vi "SeqMgr.Sequence Load, Check Lines for Sourcing Other Files.vi"(7 "Search Folders":path[](array[path]), 8 "error in (no error)":errorcluster, 10 "Parent Scripts":path[](array[path]), 11 "Lines In":string[](array[string])) -> (0 "error out":errorcluster, 3 "Lines Out":string[](array[string]))   [LabVIEW 2024, in "EQMF.lvlib" / "SeqMgr.lvlib"]
uses:
  SeqMgr.lvlib
  <vilib>/Utility/error.llb/Trim Whitespace One-Sided.vi
  Files/File Utils.lvlib
  Strings/String Utils.lvlib
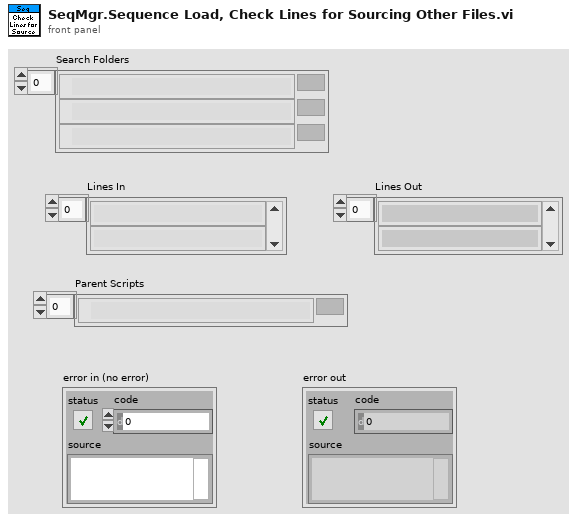
[diagram p1: front panel]
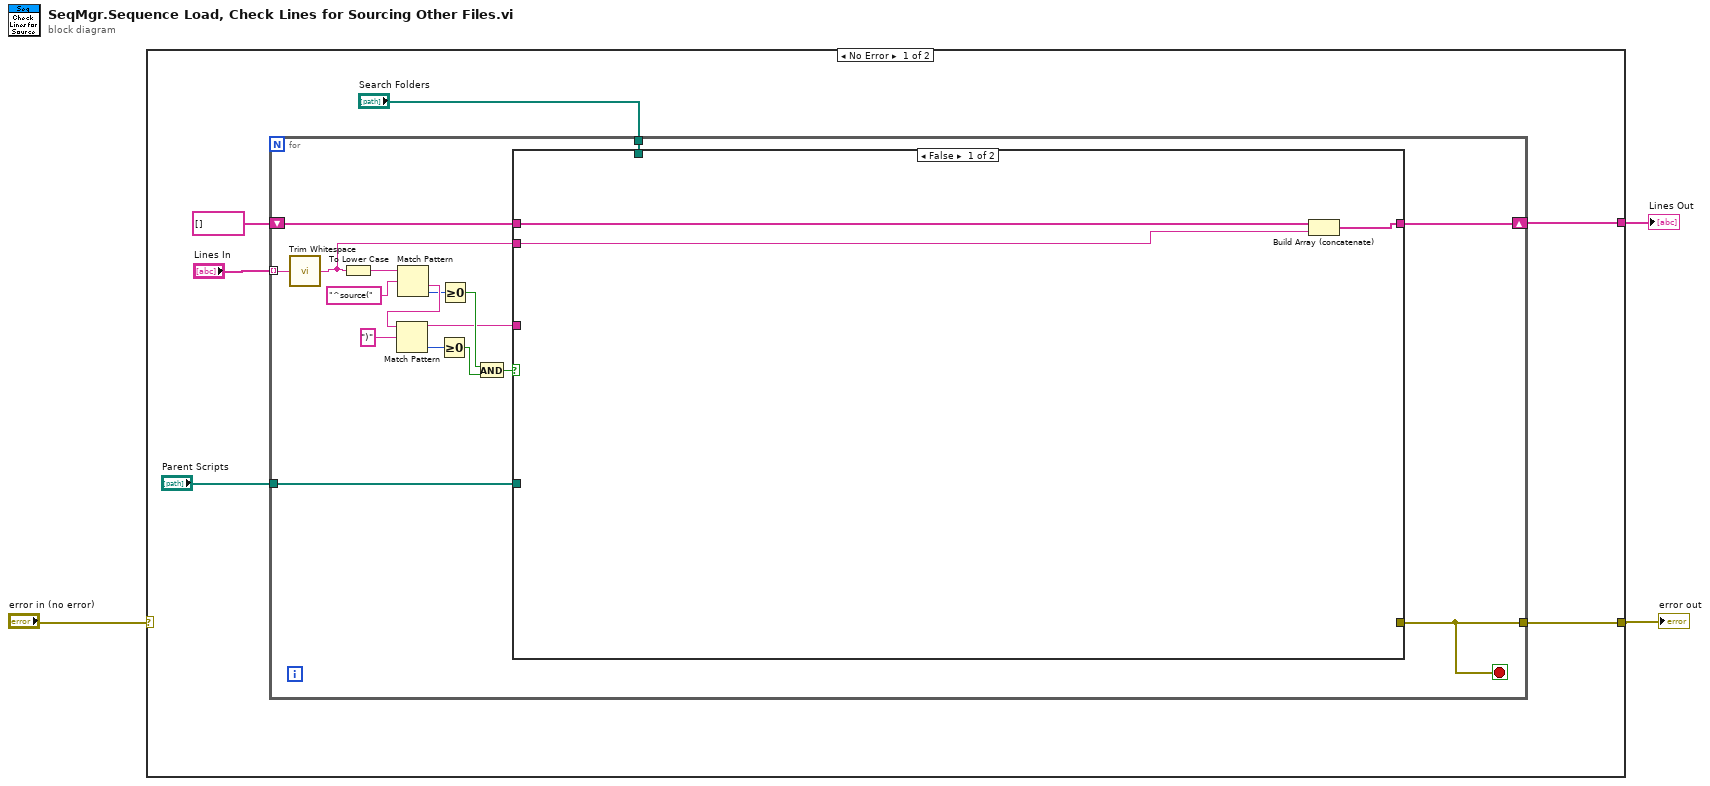
[diagram p0: block diagram]
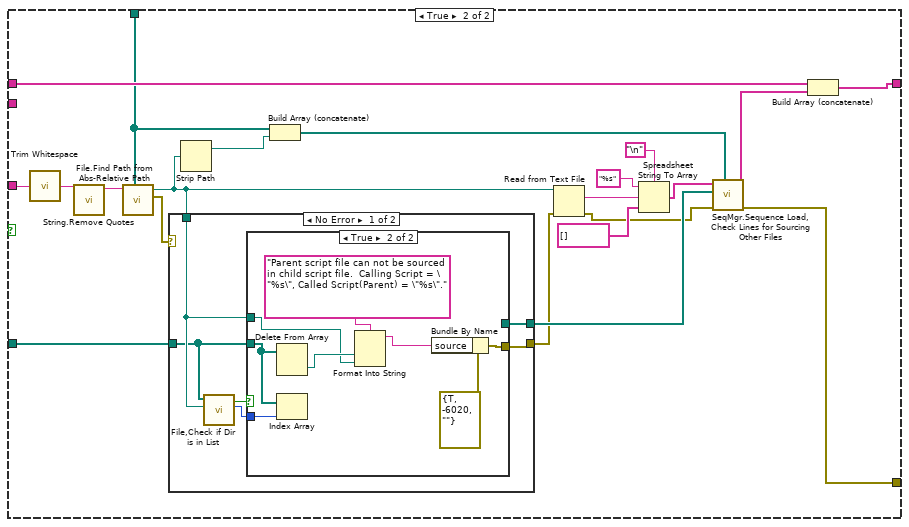
[diagram p2: hidden frame]
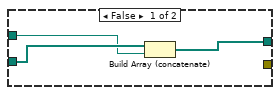
[diagram p3: hidden frame]
diagram:
  n1 = case shown="No Error" "error in (no error)" {
    selector: "error in (no error)" -> [_ w69]
    tunnel: [w6 _] -> w3
    tunnel: [w5 w69] -> w2
    frame No Error {
      n2 = for {
        tunnel: "Lines In" -> [w11] mode=indexing
        shift-right: [w16] -> w6
        shift-left: string[] [] -> [w17]
        tunnel: "Search Folders" -> [w14]
        tunnel: [w13] -> w5
        tunnel: "Parent Scripts" -> [w12]
        stop <- w13 stop-if-true
        n3 = call <vilib>:"Trim Whitespace.vi"("string"=w11) -> ("trimmed string"=w10:string)  [unwired: 1 in]
        n4 = To Lower Case(string=w10) -> (all lower case string=w25:string)
        n5 = Match Pattern(string=w25, regular expression="^source(") -> (after substring=w24:string, offset past match=w22:i32)  [unwired: 1 in, 2 out]
        n6 = Match Pattern(string=w24, regular expression=")") -> (before substring=w15:string, offset past match=w21:i32)  [unwired: 1 in, 2 out]
        n7 = Greater Or Equal To 0?(x=w21) -> (x >= 0?=w19:bool)
        n8 = Greater Or Equal To 0?(x=w22) -> (x >= 0?=w20:bool)
        n9 = And(x=w20, y=w19) -> (x .and. y?=w18:bool)
        n10 = case shown="False" w18 {
          tunnel: w17 -> [w29 w50]
          tunnel: [w28 w49] -> w16
          tunnel: w10 -> [w27 _]
          tunnel: w15 -> [_ w48]
          tunnel: w14 -> [_ w33]
          tunnel: [_ w41] -> w13
          tunnel: w12 -> [_ w40]
          frame False {
            n11 = Build Array (concatenate)(w29, w27) -> (w28:string[])
          }
          frame True {
            n12 = call <vilib>:"Trim Whitespace.vi"("string"=w48) -> ("trimmed string"=w31:string)  [unwired: 1 in]
            n13 = call "String.Remove Quotes.vi"("String With Quotes"=w31) -> ("String No Quotes"=w30:string)  [unwired: 9 in, 1 out]
            n14 = call "File.Find Path from Abs-Relative Path.vi"("Search Folders"=w33, "Rel Path"=w30) -> ("error out"=w39:errorcluster, "Path"=w35:path)  [unwired: 8 in]
            n15 = case shown="No Error" w39 {
              selector: w39 -> [_ w68]
              tunnel: w35 -> [w55 _]
              tunnel: w40 -> [w54 _]
              tunnel: [w51 w68] -> w37
              tunnel: [w53 _] -> w38
              frame No Error {
                n16 = call "File,Check if Dir is in List.vi"("Path"=w55, "List of Paths"=w54) -> ("Index"=w52:i32, "In List"=w56:bool)  [unwired: 8 in]
                n17 = case shown="True" w56 {
                  tunnel: w55 -> [w57 w60]
                  tunnel: w54 -> [w59 w66]
                  tunnel: [w58 _] -> w53
                  tunnel: w52 -> [_ w67]
                  tunnel: [_ w65] -> w51
                  frame False {
                    n18 = Build Array (concatenate)(w59, w57) -> (w58:path[])
                  }
                  frame True {
                    n19 = Delete From Array(array=w66) -> (deleted portion=w62:path)  [unwired: 2 in, 1 out]
                    n20 = Index Array(array=w66, index=w67) -> ()  [unwired: 1 out]
                    n21 = Format Into String(format string="Parent script file can not be sourced in child script file.  Calling Script = \"%s\", Called Script(Parent) = \"%s\".", w62, w60) -> (resulting string=w61:string)  [unwired: 2 in, 1 out]
                    n22 = Bundle By Name(cluster=errorcluster {"status"=TRUE, "code"=-6020, "source"=""} ("error constant"), "source"=w61) -> (w65:errorcluster)
                  }
                }
              }
              frame Error {
              }
            }
            n23 = Strip Path(path=w35) -> (stripped path=w34:path)  [unwired: 1 out]
            n24 = Build Array (concatenate)(w33, w34) -> (w32:path[])
            n25 = Read from Text File(file (use dialog)=w35, error in=w37) -> (text=w44:string, error out=w36:errorcluster)  [unwired: 2 in, 2 out]
            n26 = Spreadsheet String To Array(delimiter (Tab)="\n", format string="%s", spreadsheet string=w44, array type (2D Dbl)=string[] []) -> (array=w43:string[])
            n27 = call "SeqMgr.Sequence Load, Check Lines for Sourcing Other Files.vi"("Search Folders"=w32, "error in (no error)"=w36, "Parent Scripts"=w38, "Lines In"=w43) -> ("error out"=w41:errorcluster, "Lines Out"=w42:string[])  [unwired: 6 in]
            n28 = Build Array (concatenate)(w50, w42) -> (w49:string[])
          }
        }
      }
    }
    frame Error {
    }
  }
  "Lines Out" <- w3
  "error out" <- w2
